vi "Set_Field_AMI.vi"() -> ()   [LabVIEW 2018]
uses:
  Configurations/AMI_cluster.ctl
  Global/Global Variables/Data_Display_global.vi
  Global/Global Variables/global.vi
panel:
  out "AMI_Cluster":T1={"Y Axis Status"=enum."RAMPING", "Z Axis Status"=enum."RAMPING", "Y-Axis (T)"=0.0, "Y-Axis Setpoint (T)"=0.0, "Y-Axis Rate (T/min)"=0.0, "Z-Axis (T)"=0.0, "Z-Axis Setpoint (T)"=0.0, "Z-Axis Rate (T/min)"=0.0, "B AMI rate (T)"=0.0, "AMI Monitor"=FALSE, "AMI Set field rates"=FALSE, "AMI Set field"=FALSE, "Switch Heater Y"=FALSE, "Switch Heater Z"=FALSE, "Switch Heater On"=FALSE, "B AMI (T)"=0.0, "B AMI Setpoint (T)"=0.0, "Phi AMI (Deg) "=0.0, "Phi AMI Setpoint (Deg) "=0.0}
  in  "Cancel Button":bool
  in  "OK Button":bool
  in  "Rate":dbl
  in  "AMI Setpoint Phi(Deg)":dbl
  in  "AMI Setpoint B(T)":dbl
  # "AMI-Cluster"
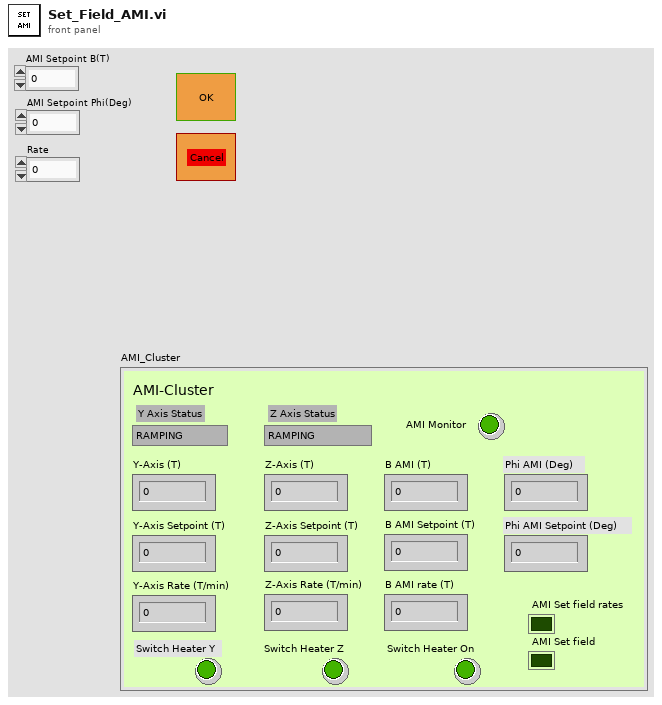
[diagram p1: front panel]
types:
  T1 = typedef "AMI_cluster.ctl" = cluster{"Y Axis Status":enum16{"", "RAMPING", "HOLDING", "PAUSED", "MANUAL UP", "MANUAL DOWN", "ZEROING CURRENT", "QUENCH DETECTED", "HEATING SWITCH", "AT ZER0", "COOLING SWITCH"}, "Z Axis Status":enum16{"", "RAMPING", "HOLDING", "PAUSED", "MANUAL UP", "MANUAL DOWN", "ZEROING CURRENT", "QUENCH DETECTED", "HEATING SWITCH", "AT ZER0", "COOLING SWITCH"}, "Y-Axis (T)":dbl, "Y-Axis Setpoint (T)":dbl, "Y-Axis Rate (T/min)":dbl, "Z-Axis (T)":dbl, "Z-Axis Setpoint (T)":dbl, "Z-Axis Rate (T/min)":dbl, "B AMI rate (T)":dbl, "AMI Monitor":bool, "AMI Set field rates":bool, "AMI Set field":bool, "Switch Heater Y":bool, "Switch Heater Z":bool, "Switch Heater On":bool, "B AMI (T)":dbl, "B AMI Setpoint (T)":dbl, "Phi AMI (Deg) ":dbl, "Phi AMI Setpoint (Deg) ":dbl}
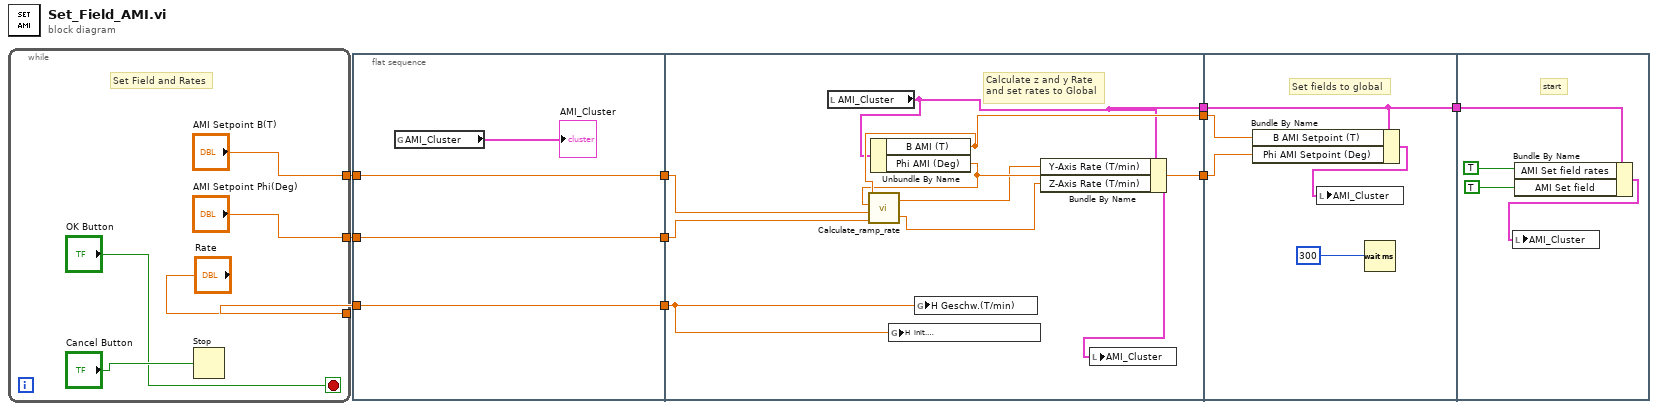
[diagram p0: block diagram]
diagram:
  n1 = while {
    tunnel: ["AMI Setpoint B(T)"] -> w10
    tunnel: ["AMI Setpoint Phi(Deg)"] -> w9
    tunnel: ["Rate"] -> w8
    stop <- "OK Button" stop-if-true
    # "Set Field and Rates"
    n2 = Stop(stop? (T)="Cancel Button") -> ()
  }
  n3 = flat-sequence {
    tunnel: w8 -> [w17]
    tunnel: w9 -> [w18]
    tunnel: w10 -> [w19]
    tunnel: [w19] -> w5
    tunnel: [w18] -> w4
    tunnel: [w17] -> w3
    tunnel: [w25] -> w7
    tunnel: [w24] -> w6
    tunnel: w5 -> [w28]
    tunnel: w4 -> [w27]
    tunnel: w3 -> [w26]
    tunnel: [w21] -> w2
    tunnel: w7 -> [w29]
    tunnel: w6 -> [w30]
    tunnel: w2 -> [w32]
    tunnel: [w32] -> w1
    tunnel: w1 -> [w37]
    frame #0 {
      n4 = global read "Data_Display_global.vi" "AMI_Cluster"() -> (→"AMI_Cluster":T1)
    }
    frame #1 {
      # "Calculate z and y Rate\nand set rates to Global"
      n5 = local read "AMI_Cluster"() -> (w21:T1)
      n6 = Unbundle By Name(w21) -> ("B AMI (T)"=w25:dbl, "Phi AMI (Deg)"=w24:dbl)
      n7 = call "Calculate_ramp_rate.vi"("Phi (Deg)"=w27, "H_final (T)"=w28, "Phi_init (Deg)"=w24, "H_init (T)"=w25) -> ("Z-Ramp"=w22:dbl, "Y-Ramp"=w23:dbl)  [unwired: 2 in]
      n8 = global write "global.vi" "H  init. \nGeschw.(T/min)"(w26) -> ()
      n9 = global write "global.vi" "H Geschw.(T/min)"(w26) -> ()
      n10 = Bundle By Name(cluster=w21, "Y-Axis Rate (T/min)"=w23, "Z-Axis Rate (T/min)"=w22) -> (w20:T1)
      n11 = local write "AMI_Cluster"(w20) -> ()
    }
    frame #2 {
      # "Set fields to global"
      n12 = Bundle By Name(cluster=w32, "B AMI Setpoint (T)"=w29, "Phi AMI Setpoint (Deg)"=w30) -> (w31:T1)
      n13 = local write "AMI_Cluster"(w31) -> ()
      n14 = Wait (ms)(milliseconds to wait=300) -> ()  [unwired: 1 out]
    }
    frame #3 {
      # "start"
      n15 = Bundle By Name(cluster=w37, "AMI Set field rates"=TRUE, "AMI Set field"=TRUE) -> (w36:T1)
      n16 = local write "AMI_Cluster"(w36) -> ()
    }
  }
